vi "Test Switch Tables.vi"() -> ()   [LabVIEW 2019, in "LV-Data.PGSQL.lvclass"]
uses:
  LV-Data.PGSQL.lvclass
  LV-Data/Typedefs/Operation--enum.ctl
  <vilib>/addons/_JKI Toolkits/Caraya/classes/Assert/Assert Not Error.vi
  <vilib>/addons/_JKI Toolkits/Caraya/classes/Test/Test.lvclass
  LV-Data/LV-Data.lvclass
  <vilib>/addons/_JKI Toolkits/Caraya/classes/Assert/Assert.lvclass
panel:
  in  "LV-Data.PG":refnum<class "LV-Data.PGSQL.lvclass">
  in  "error in (no error)":errorcluster
  out "error out":errorcluster
  out "LV-Data.PG out":refnum<class "LV-Data.PGSQL.lvclass">
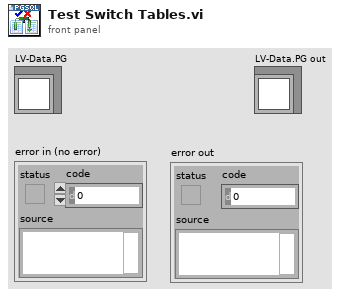
[diagram p1: front panel]
types:
  T1 = typedef "LV-Data.lvclass/Operation--enum.ctl" = enum16{"Read", "Write", "Write + Append"}
  T2 = cluster{"Column Name":string, "seconds since 1Jan1904":timestamp}
  T3 = typedef "LV-Data.PGSQL.lvclass/Datatypes--enum.ctl" = enum16{"double", "string", "integer", "boolean"}
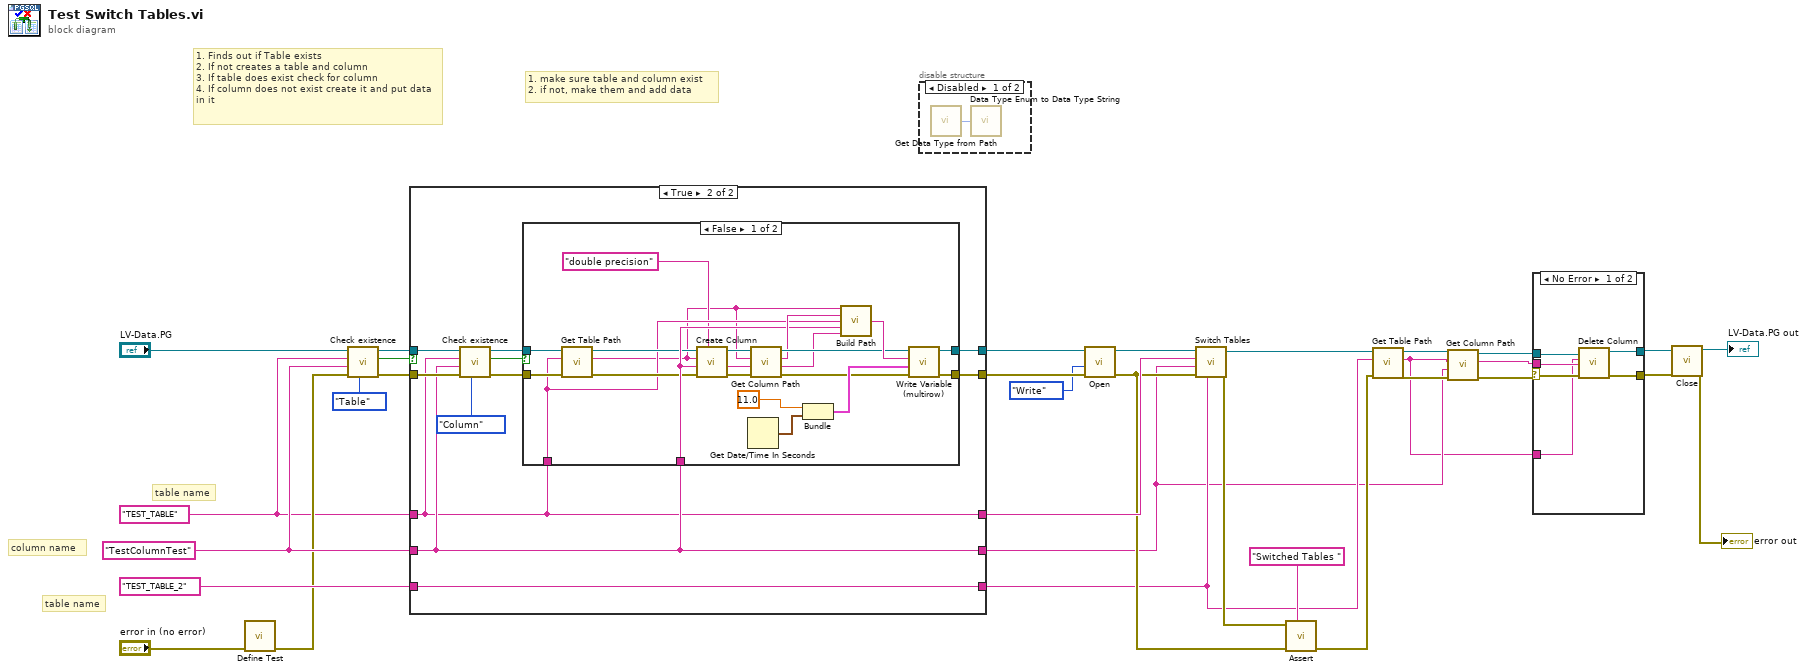
[diagram p0: block diagram]
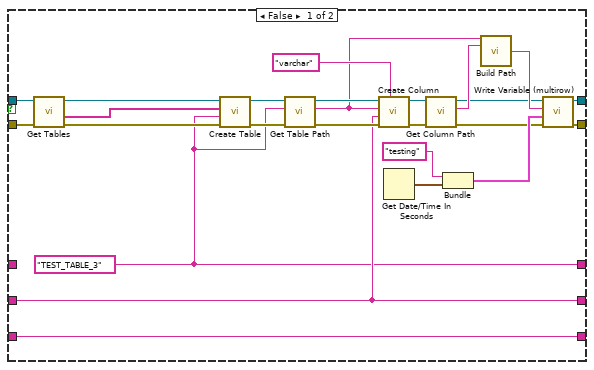
[diagram p3: hidden frame]
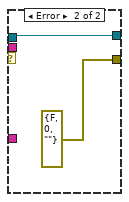
[diagram p5: hidden frame]
diagram:
  w30 = "TestColumnTest" ("Column Name")
  w11 = "TEST_TABLE" ("Old Table")
  # "column name"
  # "table name"
  # "table name"
  # "1. Finds out if Table exists \n2. If not creates a table and column \n3. If table does exist check for column\n4. If column does not exist create it and put data in it"
  # "1. make sure table and column exist\n2. if not, make them and add data"
  n1 = call <vilib>:"Define Test.vi"("error in (no error)"="error in (no error)") -> ("error out"=w28:errorcluster)  [unwired: 10 in]
  n2 = call "Check existence.vi"("Type"=enum16{"Column & Table", "Table", "Column"}."Table", "error in (no error)"=w28, "Column Name"=w30, "Table Name"=w11, "Data.PG"="LV-Data.PG") -> ("error out"=w20:errorcluster, "Exists?"=w22:bool, "Data.PG out"=w21:refnum<class "LV-Data.PGSQL.lvclass">)  [unwired: 4 in]
  n3 = case shown="True" w22 {
    tunnel: [w42 w58] -> w31
    tunnel: w30 -> [w44 w61]
    tunnel: [w44 w61] -> w2
    tunnel: [w43 w60] -> w10
    tunnel: "TEST_TABLE_2" ("New Table") -> [w43 w60]
    tunnel: w21 -> [w57 w68]
    tunnel: w20 -> [w53 w67]
    tunnel: [w50 w64] -> w26
    tunnel: [w49 w62] -> w25
    tunnel: w11 -> [_ w58]
    frame False {
      w42 = "TEST_TABLE_3"
      n4 = call "Get Tables.vi"("error in (no error)"=w53, "Data.PG"=w57) -> ("error out"=w54:errorcluster, "Table Paths"=w55:string[], "Data.PG out"=w56:refnum<class "LV-Data.PGSQL.lvclass">)  [unwired: 6 in, 1 out]
      n5 = call "Create Table.vi"("error in (no error)"=w54, "New Table Name"=w42, "Table Paths"=w55, "Data.PGSQL in"=w56) -> ("error out"=w47:errorcluster, "Data.PGSQL out"=w48:refnum<class "LV-Data.PGSQL.lvclass">)  [unwired: 6 in]
      n6 = call "Get Table Path.vi"("error in (no error)"=w47, "Table Name"=w42, "Data.PG"=w48) -> ("error out"=w45:errorcluster, "Table Path"=w38:string, "Data.PG out"=w46:refnum<class "LV-Data.PGSQL.lvclass">)  [unwired: 5 in, 1 out]
      n7 = call "Create Column.vi"("new column data type"="varchar", "error in (no error)"=w45, "new column name"=w44, "selected table path"=w38, "Data.PGSQL in"=w46) -> ("error out"=w37:errorcluster, "Data.PGSQL out"=w36:refnum<class "LV-Data.PGSQL.lvclass">)  [unwired: 5 in]
      n8 = Get Date/Time In Seconds() -> (seconds since 1Jan1904=w52:timestamp)
      n9 = call "Get Column Path.vi"("error in (no error)"=w37, "Data.PG in"=w36) -> ("error out"=w34:errorcluster, "Column Path"=w35:string, "Data.PG out"=w33:refnum<class "LV-Data.PGSQL.lvclass">)  [unwired: 6 in, 1 out]
      n10 = Bundle("Column Name"="testing", "seconds since 1Jan1904"=w52) -> (w51:T2)  [unwired: 1 in]
      n11 = call "Build Path.vi"("Table path"=w38, "Column path"=w35) -> ("PG path"=w39:string)  [unwired: 13 in]
      n12 = call "Write Variable (multirow).vi"("error in (no error)"=w34, "Data"=w51, "variable"=w39, "Data.PG in"=w33) -> ("error out"=w49:errorcluster, "Data.PG out"=w50:refnum<class "LV-Data.PGSQL.lvclass">)  [unwired: 4 in, 2 out]
    }
    frame True {
      n13 = call "Check existence.vi"("Type"=enum16{"Column & Table", "Table", "Column"}."Column", "error in (no error)"=w67, "Column Name"=w61, "Table Name"=w58, "Data.PG"=w68) -> ("error out"=w63:errorcluster, "Exists?"=w66:bool, "Data.PG out"=w65:refnum<class "LV-Data.PGSQL.lvclass">)  [unwired: 4 in]
      n14 = case shown="False" w66 {
        tunnel: w65 -> [w74 w90]
        tunnel: [w86 w90] -> w64
        tunnel: w63 -> [w75 w89]
        tunnel: [w85 w89] -> w62
        tunnel: w61 -> [w77 _]
        tunnel: w58 -> [w71 _]
        frame False {
          n15 = call "Get Table Path.vi"("error in (no error)"=w75, "Table Name"=w71, "Data.PG"=w74) -> ("error out"=w73:errorcluster, "Table Path"=w69:string, "Data.PG out"=w72:refnum<class "LV-Data.PGSQL.lvclass">)  [unwired: 5 in, 1 out]
          n16 = call "Create Column.vi"("new column data type"="double precision", "error in (no error)"=w73, "new column name"=w77, "selected table path"=w69, "Data.PGSQL in"=w72) -> ("error out"=w79:errorcluster, "Data.PGSQL out"=w83:refnum<class "LV-Data.PGSQL.lvclass">)  [unwired: 5 in]
          n17 = Get Date/Time In Seconds() -> (seconds since 1Jan1904=w87:timestamp)
          n18 = call "Get Column Path.vi"("error in (no error)"=w79, "Column Name"=w77, "Table path"=w69, "Data.PG in"=w83) -> ("error out"=w78:errorcluster, "Column Unit"=w80:string, "Column Path"=w81:string, "Data.PG out"=w82:refnum<class "LV-Data.PGSQL.lvclass">)  [unwired: 4 in]
          n19 = Bundle(11.0, "seconds since 1Jan1904"=w87) -> (w88:cluster{dbl, "seconds since 1Jan1904":timestamp})  [unwired: 1 in]
          n20 = call "Build Path.vi"("Table path"=w69, "Column path"=w81, "Table name"=w71, "Column name"=w77, "Column units"=w80) -> ("PG path"=w84:string)  [unwired: 10 in]
          n21 = call "Write Variable (multirow).vi"("error in (no error)"=w78, "Data"=w88, "variable"=w84, "Data.PG in"=w82) -> ("error out"=w85:errorcluster, "Data.PG out"=w86:refnum<class "LV-Data.PGSQL.lvclass">)  [unwired: 4 in, 2 out]
        }
        frame True {
        }
      }
    }
  }
  n22 = disable-structure "Diagram Disable Structure" shown="Disabled" {
    frame Disabled {
      n23 = call "Get Data Type from Path.vi"() -> ("data type"=w91:T3)  [unwired: 1 in]
      n24 = call "Data Type Enum to Data Type String.vi"("data type"=w91) -> ()  [unwired: 1 out]
    }
    frame Enabled {
    }
  }
  n25 = call-dynamic "Open.vi"("error in (no error)"=w25, "Operation"=Operation--enum."Write", "Data.PG in"=w26) -> ("error out"=w14:errorcluster, "Data.PG out"=w15:refnum<class "LV-Data.PGSQL.lvclass">)  [unwired: 7 in]
  n26 = call "Switch Tables.vi"("New Table Name"=w10, "error in (no error)"=w14, "Column Name"=w2, "Old Table Name"=w31, "Data.PG"=w15) -> ("error out"=w13:errorcluster, "Data.PG out"=w9:refnum<class "LV-Data.PGSQL.lvclass">)  [unwired: 5 in]
  n27 = call-poly <vilib>:"Assert.vi"("Label"="Switched Tables ", "error in (no error)"=w14, "Not Error?"=w13) -> ("error out"=w3:errorcluster)  [unwired: 8 in]
  n28 = call "Get Table Path.vi"("error in (no error)"=w3, "Table Name"=w10, "Data.PG"=w9) -> ("error out"=w4:errorcluster, "Table Path"=w1:string, "Data.PG out"=w8:refnum<class "LV-Data.PGSQL.lvclass">)  [unwired: 5 in, 1 out]
  n29 = call "Get Column Path.vi"("error in (no error)"=w4, "Column Name"=w2, "Table path"=w1, "Data.PG in"=w8) -> ("error out"=w5:errorcluster, "Column Path"=w6:string, "Data.PG out"=w7:refnum<class "LV-Data.PGSQL.lvclass">)  [unwired: 4 in, 1 out]
  n30 = case shown="No Error" w5 {
    selector: w5 -> [w97 _]
    tunnel: [w96 errorcluster {"status"=FALSE, "code"=0, "source"=""} ("error out")] -> w17
    tunnel: [w95 w98] -> w18
    tunnel: w7 -> [w94 w98]
    tunnel: w6 -> [w93 _]
    tunnel: w1 -> [w92 _]
    frame No Error {
      n31 = call "Delete Column.vi"("error in"=w97, "Column path"=w93, "Table Path"=w92, "LV-Data.PG"=w94) -> ("error out"=w96:errorcluster, "LV-Data.PG out"=w95:refnum<class "LV-Data.PGSQL.lvclass">)  [unwired: 6 in]
    }
    frame Error {
    }
  }
  n32 = call-dynamic "Close.vi"("error in (no error)"=w17, "Data.PG in"=w18) -> ("error out"=→"error out":errorcluster, "Data.PG out"=→"LV-Data.PG out":refnum<class "LV-Data.PGSQL.lvclass">)  [unwired: 8 in]
